vi "Write paper data.vi"(0 "Refnum in":T1, 11 "error in (no error)":errorcluster, 12 "Names":string[](array[string]), 13 "Costs":dbl[][](array[numeric]), 14 "Days":bool[][](array[boolean])) -> (4 "Refnum out":T1, 15 "error out":errorcluster)   [LabVIEW 2015]
uses:
  <vilib>/Utility/config.llb/Config Data RefNum.ctl
  <vilib>/Utility/config.llb/Read Key (Path).vi
  <vilib>/Utility/file.llb/Write Delimited Spreadsheet (string).vi
  <vilib>/Utility/file.llb/Write Delimited Spreadsheet (DBL).vi
  <vilib>/Utility/config.llb/NI_LVConfig.lvlib
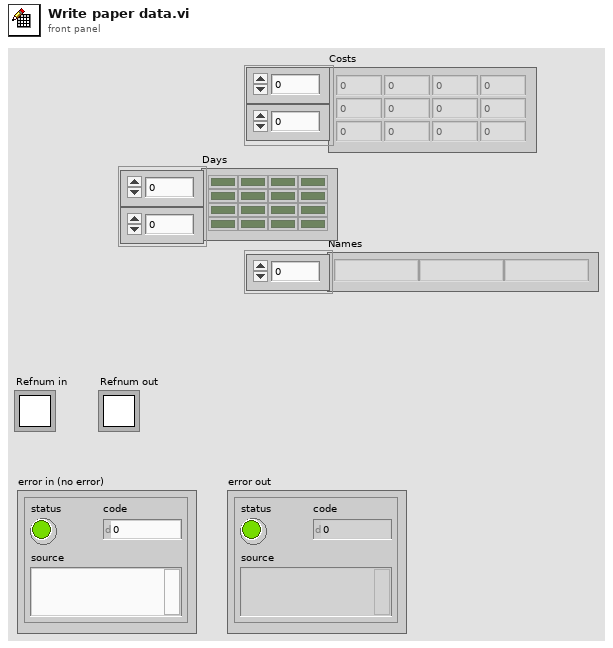
[diagram p1: front panel]
types:
  T1 = typedef "NI_LVConfig.lvlib/Config Data RefNum.ctl" = refnum<k1>
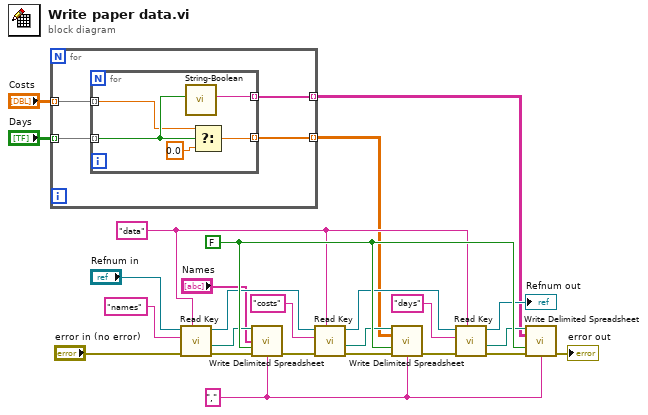
[diagram p0: block diagram]
diagram:
  w25 = FALSE ("append to file? (F)")
  w6 = "," ("delimiter (\\t)")
  w16 = "data" ("section")
  n1 = for {
    tunnel: "Days" -> [w29] mode=indexing
    tunnel: [w28] -> w3 mode=indexing
    tunnel: "Costs" -> [w27] mode=indexing
    tunnel: [w26] -> w1 mode=indexing
    n2 = for {
      tunnel: w29 -> [w33] mode=indexing
      tunnel: [w34] -> w28 mode=indexing
      tunnel: w27 -> [w32] mode=indexing
      tunnel: [w30] -> w26 mode=indexing
      n3 = call "String-Boolean.vi"("Boolean in"=w33) -> ("String out"=w34:string)  [unwired: 9 in, 1 out]
      n4 = Select(t=w32, s=w33, f=0.0) -> (s? t:f=w30:dbl)
    }
  }
  n5 = call-poly <vilib>:"Read Key.vi"("section"=w16, "error in (no error)"="error in (no error)", "key"="names", "refnum"="Refnum in") -> ("error out"=w20:errorcluster, "value"=w9:path, "refnum out"=w19:T1)  [unwired: 4 in, 1 out]
  n6 = call-poly <vilib>:"Write Delimited Spreadsheet.vi"("file path (dialog if empty)"=w9, "1D data"="Names", "append to file? (F)"=w25, "error in (no error)"=w20, "delimiter (\\t)"=w6) -> ("error out"=w12:errorcluster)  [unwired: 9 in, 1 out]
  n7 = call-poly <vilib>:"Read Key.vi"("section"=w16, "error in (no error)"=w12, "key"="costs", "refnum"=w19) -> ("error out"=w18:errorcluster, "value"=w8:path, "refnum out"=w17:T1)  [unwired: 4 in, 1 out]
  n8 = call-poly <vilib>:"Write Delimited Spreadsheet.vi"("file path (dialog if empty)"=w8, "2D data"=w1, "append to file? (F)"=w25, "error in (no error)"=w18, "delimiter (\\t)"=w6) -> ("error out"=w11:errorcluster)  [unwired: 9 in, 1 out]
  n9 = call-poly <vilib>:"Read Key.vi"("section"=w16, "error in (no error)"=w11, "key"="days", "refnum"=w17) -> ("error out"=w10:errorcluster, "value"=w7:path, "refnum out"=→"Refnum out":T1)  [unwired: 4 in, 1 out]
  n10 = call-poly <vilib>:"Write Delimited Spreadsheet.vi"("file path (dialog if empty)"=w7, "2D data"=w3, "append to file? (F)"=w25, "error in (no error)"=w10, "delimiter (\\t)"=w6) -> ("error out"=→"error out":errorcluster)  [unwired: 9 in, 1 out]
